vi "Set Multi Track H Range.vi"(10 "iEnd":i32, 11 "iStart":i32) -> (3 "function return":u32)   [LabVIEW 2018, in "AndorSDK.lvlib"]
doc: "EXPNETTYPE unsigned int WINAPI SetMultiTrackHRange(int iStart, int iEnd);"
uses:
  AndorSDK.lvlib
  ATMCD32D.dll
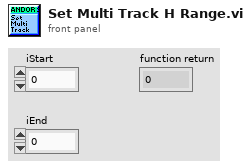
[diagram p1: front panel]
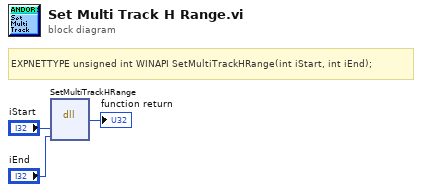
[diagram p0: block diagram]
diagram:
  # "EXPNETTYPE unsigned int WINAPI SetMultiTrackHRange(int iStart, int iEnd);"
  n1 = dll-call lib="PTH2babs E\nPersönliches02 - Arbeit03-HiwijobsLabviewCodelibANDOR\tAndor SDK\nATMCD32D.*" fn="SetMultiTrackHRange"("iStart"="iStart", "iEnd"="iEnd") -> (→"function return":u32)  [unwired: 5 in, 2 out]
